vi "generate_histogram.vi"(4 "M min":dbl, 5 "V max":dbl, 6 "V min":dbl, 7 "M max":dbl, 9 "Mass":dbl[](array[numeric]), 10 "Veloicty":dbl[](array[numeric]), 11 "dimension size":i32=100) -> (2 "Intensity Graph":dbl[][](graph), 3 "output array":dbl[][](array[numeric]))   [LabVIEW 2011]
panel:
  out "x/y":dbl
  out "min value":dbl
  out "max value":dbl
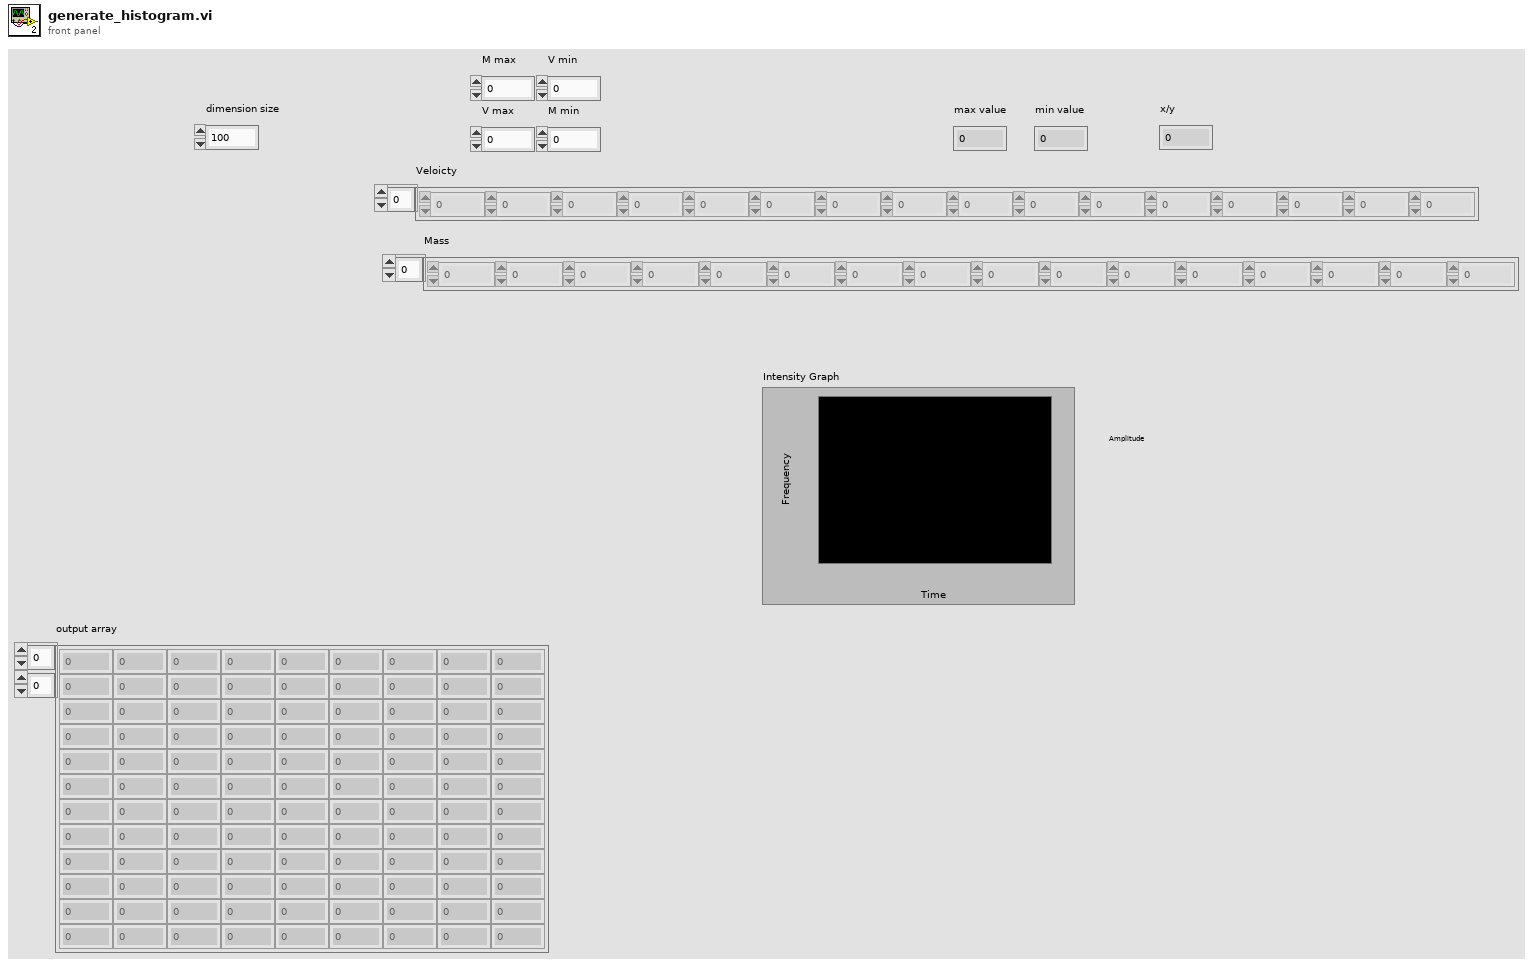
[diagram p1: front panel]
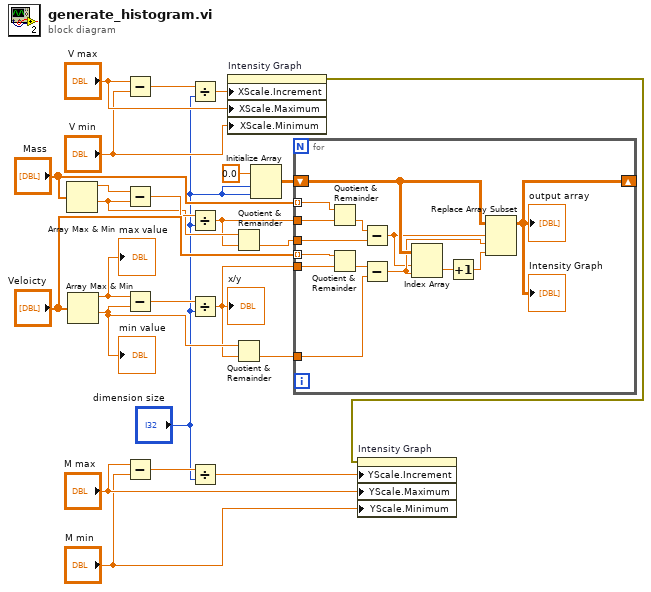
[diagram p0: block diagram]
diagram:
  n1 = Array Max & Min(array="Mass") -> (max value=w21:dbl, min value=w15:dbl)  [unwired: 2 out]
  n2 = Array Max & Min(array="Veloicty") -> (max value=w20:dbl, min value=w16:dbl)  [unwired: 2 out]
  "max value" <- w20
  "min value" <- w16
  n3 = Subtract(x="V max", y="V min") -> (x-y=w6:dbl)
  n4 = Subtract(x=w21, y=w15) -> (x-y=w19:dbl)
  n5 = Subtract(x=w20, y=w16) -> (x-y=w18:dbl)
  n6 = Subtract(x="M max", y="M min") -> (x-y=w10:dbl)
  n7 = Divide(x=w6, y="dimension size") -> (x/y=w4:dbl)
  n8 = Divide(x=w19, y="dimension size") -> (x/y=w11:dbl)
  n9 = Divide(x=w18, y="dimension size") -> (x/y=w12:dbl)
  "x/y" <- w12
  n10 = Divide(x=w10, y="dimension size") -> (x/y=w9:dbl)
  n11 = property on="Intensity Graph" class="IntGraph (strict)"("XScale.Increment"=w4, "XScale.Maximum"="V max", "XScale.Minimum"="V min") -> (error out=w1:errorcluster)  [unwired: 2 in, 1 out]
  n12 = Quotient & Remainder(x=w15, y=w11) -> (floor(x/y)=w14:dbl)  [unwired: 1 out]
  n13 = Quotient & Remainder(x=w16, y=w12) -> (floor(x/y)=w13:dbl)  [unwired: 1 out]
  n14 = Initialize Array(0.0 ("element"), "dimension size", "dimension size") -> (w24:dbl[][])
  n15 = for {
    tunnel: "Veloicty" -> [w37] mode=indexing
    tunnel: "Mass" -> [w36] mode=indexing
    shift-right: [w35] -> _
    shift-left: w24 -> [w32]
    tunnel: w11 -> [w34]
    tunnel: w12 -> [w33]
    tunnel: w13 -> [w26]
    tunnel: w14 -> [w25]
    n16 = Quotient & Remainder(x=w36, y=w34) -> (floor(x/y)=w27:dbl)  [unwired: 1 out]
    n17 = Quotient & Remainder(x=w37, y=w33) -> (floor(x/y)=w29:dbl)  [unwired: 1 out]
    n18 = Subtract(x=w27, y=w25) -> (x-y=w28:dbl)
    n19 = Subtract(x=w29, y=w26) -> (x-y=w30:dbl)
    n20 = Index Array(array=w32, index (row)=w28, index (col)=w30) -> (element=w38:dbl)
    n21 = Increment(x=w38) -> (x+1=w31:dbl)
    n22 = Replace Array Subset(array=w32, new element=w31, index (row)=w28, index (col)=w30) -> (w35:dbl[][])
    "output array" <- w35
    "Intensity Graph" <- w35
  }
  n23 = property on="Intensity Graph" class="IntGraph (strict)"(error in=w1, "YScale.Increment"=w9, "YScale.Maximum"="M max", "YScale.Minimum"="M min") -> ()  [unwired: 1 in, 2 out]
